vi "xps_panel_DO_retrieve_ftp_trajectories.vi"(8 "error in (no error)":errorcluster, 11 "newport_xps_panel in":refnum<class "newport_xps_panel.lvclass">) -> (0 "error out":errorcluster, 3 "newport_xps_panel out":refnum<class "newport_xps_panel.lvclass">)   [LabVIEW 2015, in "newport_xps_panel.lvclass"]
uses:
  newport_xps_panel.lvclass
  newport_xps/newport_xps.lvclass
  newport_xps_panel.lvclass/newport_xps_panel.ctl
  UI/panel_class/panel.lvclass
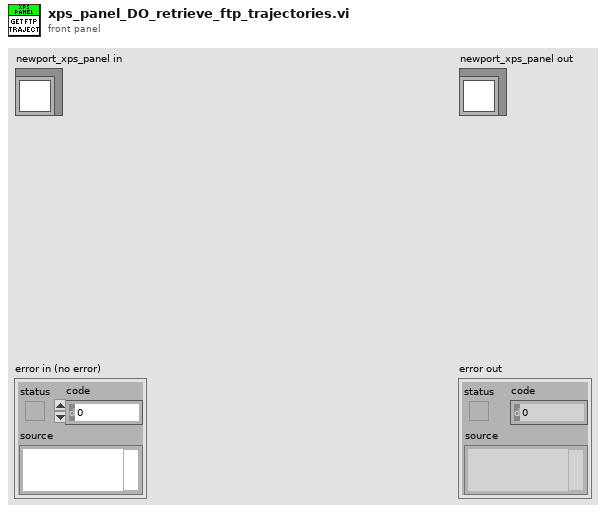
[diagram p1: front panel]
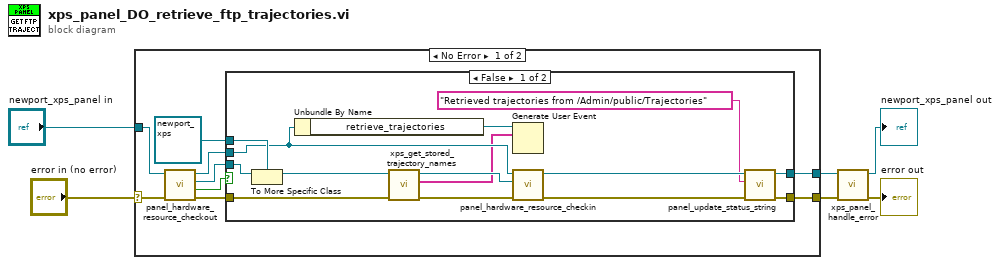
[diagram p0: block diagram]
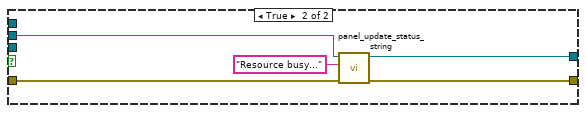
[diagram p2: hidden frame]
diagram:
  n1 = case shown="No Error" "error in (no error)" {
    selector: "error in (no error)" -> [w15 w36]
    tunnel: [w9 w36] -> w4
    tunnel: [w8 w35] -> w2
    tunnel: "newport_xps_panel in" -> [w14 w35]
    frame No Error {
      n2 = call "panel_hardware_resource_checkout.vi"("error in (no error)"=w15, "panel in"=w14) -> ("error out"=w10:errorcluster, "timed out?"=w13:bool, "hardware.lvclass"=w11:refnum<class "hardware.lvclass">, "panel out"=w12:refnum<class "newport_xps_panel.lvclass">)  [unwired: 6 in]
      n3 = case shown="False" w13 {
        tunnel: w12 -> [w19 w31]
        tunnel: w11 -> [w29 _]
        tunnel: w10 -> [w22 w34]
        tunnel: [w25 w33] -> w9
        tunnel: [w24 w30] -> w8
        tunnel: refnum<class "newport_xps.lvclass"> refnum ("newport_xps in") -> [w28 _]
        frame False {
          n4 = To More Specific Class(target class=w28, reference=w29) -> (specific class reference=w23:refnum<class "newport_xps.lvclass">)  [unwired: 1 in, 1 out]
          n5 = Unbundle By Name(w19) -> ("retrieve_trajectories"=w18:refnum<user-event>)
          n6 = call "xps_get_stored_trajectory_names.vi"("error in (no error)"=w22, "newport_xps in"=w23) -> ("error out"=w20:errorcluster, "trajectory_names"=w17:string[], "newport_xps out"=w21:refnum<class "newport_xps.lvclass">)  [unwired: 7 in]
          n7 = Generate User Event(user event=w18, event data cluster=w17) -> ()  [unwired: 2 in, 2 out]
          n8 = call "panel_hardware_resource_checkin.vi"("error in (no error)"=w20, "hardware.lvclass"=w21, "panel in"=w19) -> ("error out"=w27:errorcluster, "panel out"=w26:refnum<class "newport_xps_panel.lvclass">)  [unwired: 7 in]
          n9 = call-dynamic "panel_update_status_string.vi"("error in (no error)"=w27, "String"="Retrieved trajectories from /Admin/public/Trajectories", "newport_xps_panel in"=w26) -> ("error out"=w25:errorcluster, "newport_xps_panel out"=w24:refnum<class "newport_xps_panel.lvclass">)  [unwired: 7 in]
        }
        frame True {
          n10 = call-dynamic "panel_update_status_string.vi"("error in (no error)"=w34, "String"="Resource busy...", "newport_xps_panel in"=w31) -> ("error out"=w33:errorcluster, "newport_xps_panel out"=w30:refnum<class "newport_xps_panel.lvclass">)  [unwired: 7 in]
        }
      }
    }
    frame Error {
    }
  }
  n11 = call "xps_panel_handle_error.vi"("error in (no error)"=w4, "newport_xps_panel in"=w2) -> ("error out"=→"error out":errorcluster, "newport_xps_panel out"=→"newport_xps_panel out":refnum<class "newport_xps_panel.lvclass">)  [unwired: 8 in]
